vi "Clase7.vi"() -> ()   [LabVIEW 2011]
panel:
  out "Menor":dbl
  out "Mayor":dbl
  out "Promedio":dbl
  out "Temperatura":i32(slide) scale=0.0..100.0
  # "Generar (10 temperaturas) y al final presentar la temperatura mayor, menor y la temperatura promedio"
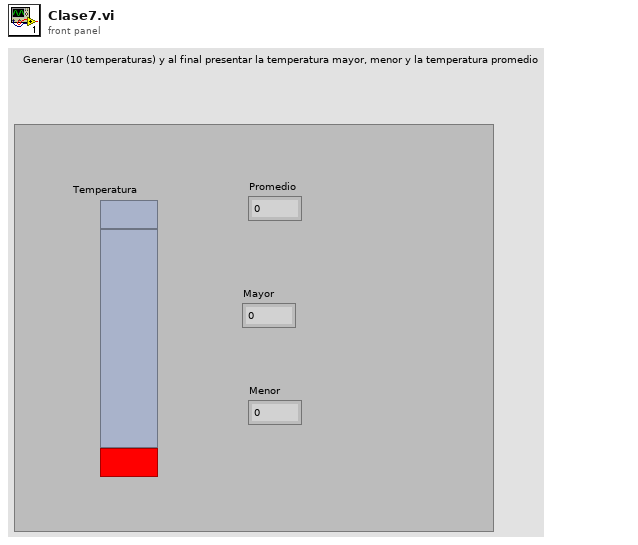
[diagram p1: front panel]
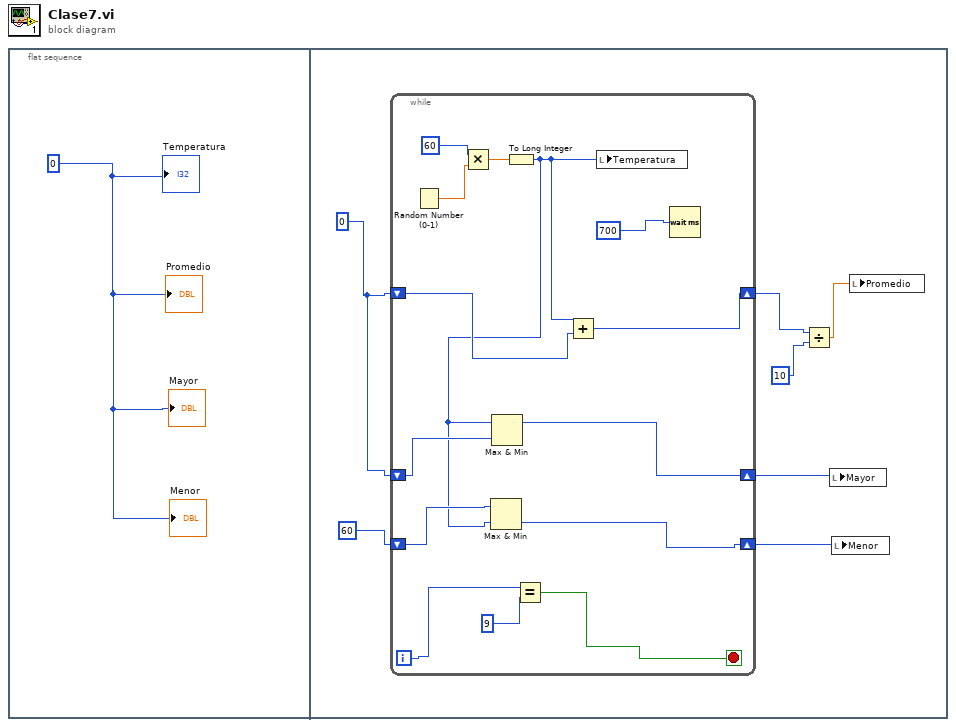
[diagram p0: block diagram]
diagram:
  n1 = flat-sequence {
    frame #0 {
      w1 = 0
      "Temperatura" <- w1
      "Promedio" <- w1
      "Mayor" <- w1
      "Menor" <- w1
    }
    frame #1 {
      w4 = 0
      n2 = while {
        shift-right: [w15] -> w8
        shift-left: w4 -> [w16]
        shift-right: [w12] -> w5
        shift-left: w4 -> [w13]
        shift-right: [w9] -> w3
        shift-left: 60 -> [w11]
        i -> [w21]
        stop <- w20 stop-if-true
        n3 = Random Number (0-1)() -> (number: 0 to 1=w17:dbl)
        n4 = Multiply(x=60, y=w17) -> (x*y=w19:dbl)
        n5 = To Long Integer(number=w19) -> (32bit integer=w10:i32)
        n6 = Max & Min(x=w11, y=w10) -> (min(x,y)=w9:i32)  [unwired: 1 out]
        n7 = Max & Min(x=w10, y=w13) -> (max(x,y)=w12:i32)  [unwired: 1 out]
        n8 = Equal?(x=w21, y=9) -> (x = y?=w20:bool)
        n9 = Add(x=w10, y=w16) -> (x+y=w15:i32)
        n10 = local write "Temperatura"(w10) -> ()
        n11 = Wait (ms)(milliseconds to wait=700) -> ()  [unwired: 1 out]
      }
      n12 = Divide(x=w8, y=10) -> (x/y=w6:dbl)
      n13 = local write "Mayor"(w5) -> ()
      n14 = local write "Menor"(w3) -> ()
      n15 = local write "Promedio"(w6) -> ()
    }
  }
